vi "OcsReadListTxtToExcel.vi"() -> ()   [LabVIEW 2011]
panel:
  out "element":i32
  out "array":string[][](array[string])
  in  ".txt":path
  out "Out":string
  in  "opname":string(combo)="FCT1"
  out "Start Time":dbl
  out "Sec":dbl
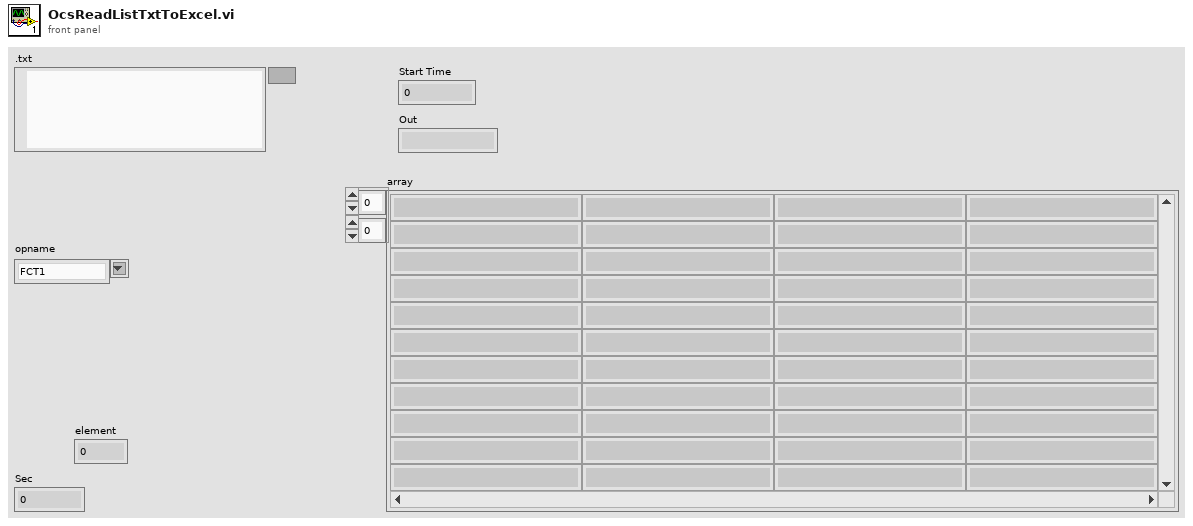
[diagram p1: front panel]
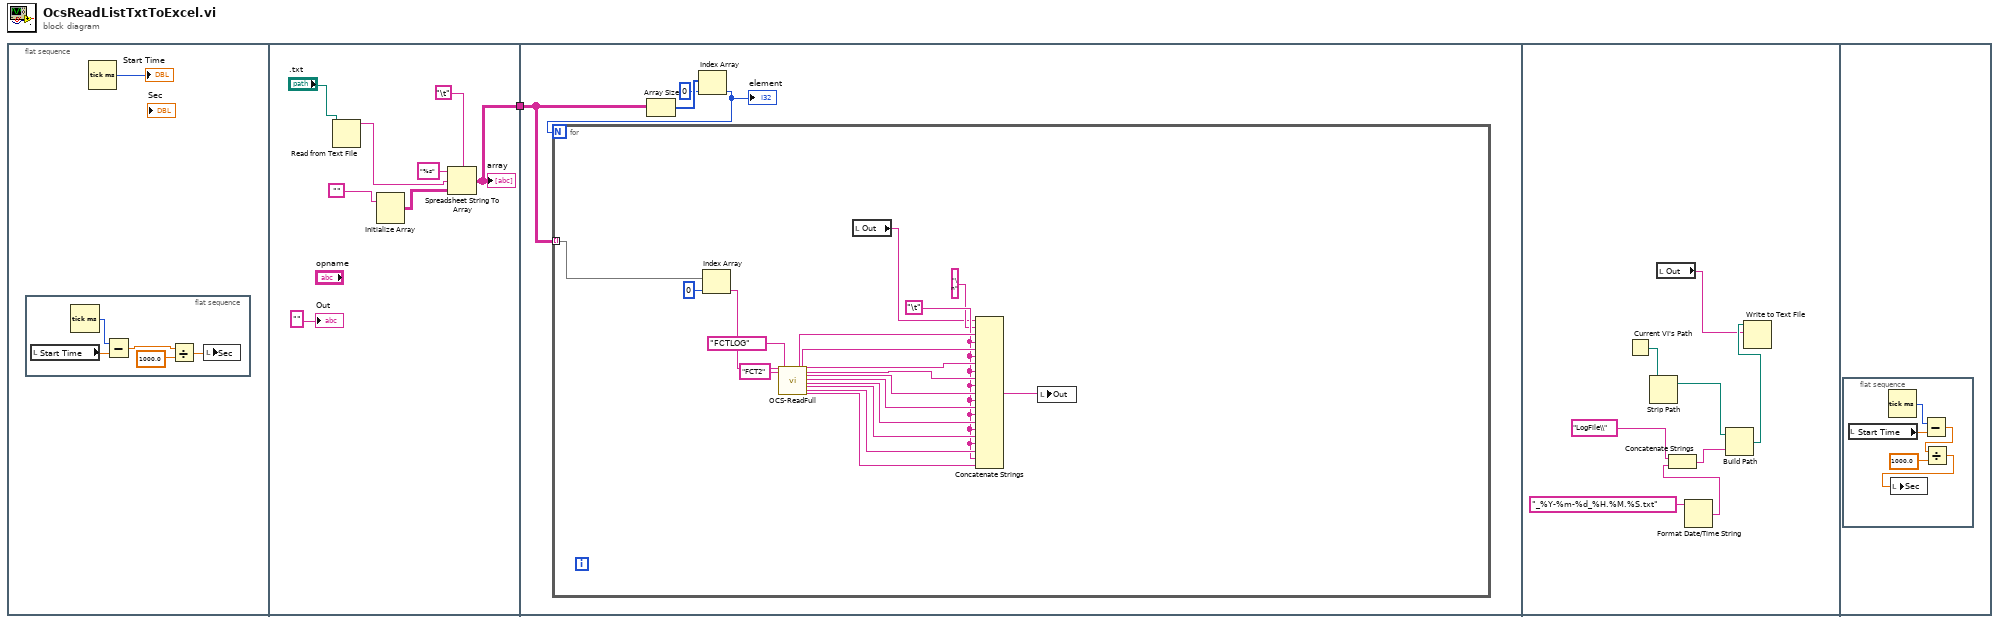
[diagram p0: block diagram]
diagram:
  n1 = flat-sequence {
    tunnel: [w9] -> w1
    tunnel: w1 -> [w16]
    frame #0 {
      n2 = flat-sequence {
        frame #0 {
          n3 = local read "Start Time"() -> (w6:dbl)
          n4 = Tick Count (ms)() -> (millisecond timer value=w7:u32)
          n5 = Subtract(x=w7, y=w6) -> (x-y=w5:dbl)
          n6 = Divide(x=w5, y=1000.0) -> (x/y=w3:dbl)
          n7 = local write "Sec"(w3) -> ()
        }
      }
      n8 = Tick Count (ms)() -> (millisecond timer value=→"Start Time":u32)
    }
    frame #1 {
      n9 = Read from Text File(file (use dialog)=".txt") -> (text=w15:string)  [unwired: 3 in, 3 out]
      n10 = Initialize Array("") -> (w14:string[][])  [unwired: 2 in]
      n11 = Spreadsheet String To Array(delimiter (Tab)="\t", format string="%s", spreadsheet string=w15, array type (2D Dbl)=w14) -> (array=w9:string[][])
      "array" <- w9
      "Out" <- ""
    }
    frame #2 {
      n12 = Array Size(array=w16) -> (size(s)=w19:i32[])
      n13 = Index Array(array=w19, index=0) -> (element=w17:i32)
      "element" <- w17
      n14 = for {
        N: w17 -> [_]
        tunnel: w16 -> [w38] mode=indexing
        w24 = "\t"
        n15 = Index Array(array=w38, index=0) -> (element=w36:string)
        n16 = call "OCS-ReadFull.vi"("SN"=w36, "OPNAME Befor"="FCT2", "TebelLogBefor"="FCTLOG") -> ("R1"=w33:string, "R2"=w32:string, "R3"=w31:string, "R4"=w30:string, "R5 SNPcb"=w29:string, "R6 SN BottomCase"=w28:string, "R7"=w27:string, "R8"=w26:string, "R9"=w25:string, "R10"=w23:string)  [unwired: 13 in, 2 out]
        n17 = local read "Out"() -> (w21:string)
        n18 = Concatenate Strings(w21, "\n" ("string"), w33, w24, w32, w24, w31, w24, w30, w24, w29, w24, w28, w24, w27, w24, w26, w24, w25, w24, w23) -> (w20:string)
        n19 = local write "Out"(w20) -> ()
      }
    }
    frame #3 {
      n20 = Current VI's Path() -> (path=w46:path)
      n21 = Strip Path(path=w46) -> (stripped path=w45:path)  [unwired: 1 out]
      n22 = local read "Out"() -> (w40:string)
      n23 = Format Date/Time String(time format string (%c)="_%Y-%m-%d_%H.%M.%S.txt") -> (date/time string=w42:string)  [unwired: 2 in]
      n24 = Concatenate Strings("LogFile\\" ("name or relative path"), w42) -> (w43:string)
      n25 = Build Path(base path=w45, name or relative path=w43) -> (appended path=w41:path)
      n26 = Write to Text File(file (use dialog)=w41, text=w40) -> ()  [unwired: 2 in, 3 out]
    }
    frame #4 {
      n27 = flat-sequence {
        frame #0 {
          n28 = local read "Start Time"() -> (w50:dbl)
          n29 = Tick Count (ms)() -> (millisecond timer value=w51:u32)
          n30 = Subtract(x=w51, y=w50) -> (x-y=w49:dbl)
          n31 = Divide(x=w49, y=1000.0) -> (x/y=w47:dbl)
          n32 = local write "Sec"(w47) -> ()
        }
      }
    }
  }
